vi "数采仪日志报警存储(子VI).vi"   [LabVIEW 2016]
types:
  T1 = cluster{"时间标识":timestamp, "设备":string, "日志信息":string, "流程参数":string}
  T2 = cluster{"时间标识":timestamp, "设备":string, "日志信息":string}
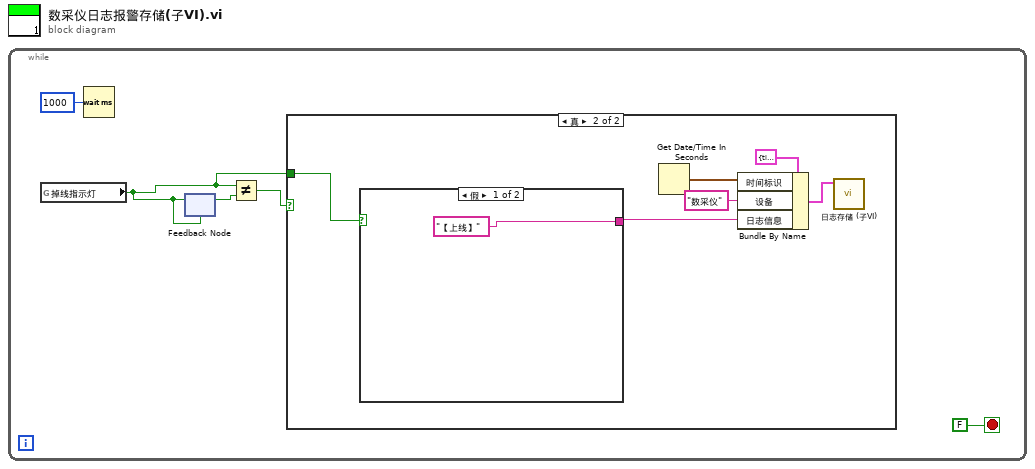
[diagram p0: block diagram]
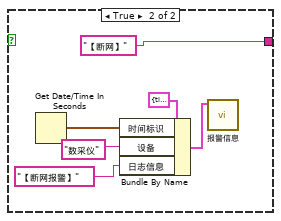
[diagram p3: hidden frame]
diagram:
  n1 = while {
    stop <- FALSE stop-if-true
    n2 = global read "全局 数据发送重叠.vi" "掉线指示灯"() -> (w1:bool)
    n3 = Wait (ms)(milliseconds to wait=u32 1000 ("等待时间（毫秒）")) -> ()  [unwired: 1 out]
    n4 = feedback-in #1(w1) -> ()
    n5 = feedback #1(w1) -> (w3:bool)
    n6 = Not Equal?(x=w1, y=w3) -> (x != y?=w2:bool)
    n7 = case shown="真" w2 {
      tunnel: w1 -> [_ w6]
      frame False {
      }
      frame True {
        n8 = case shown="假" w6 {
          tunnel: ["【上线】" ("设备") "【断网】" ("设备")] -> w7
          frame False {
          }
          frame True {
            n9 = Get Date/Time In Seconds() -> (seconds since 1Jan1904=w15:timestamp)
            n10 = Bundle By Name(cluster=T2 {"时间标识"=timestamp(0 s since 1904-01-01), "设备"="", "日志信息"=""} ("data in"), "时间标识"=w15, "设备"="数采仪", "日志信息"="【断网报警】" ("设备")) -> (w16:T2)
            n11 = call "报警信息.vi"("data in"=w16) -> ()  [unwired: 10 in, 1 out]
          }
        }
        n12 = Get Date/Time In Seconds() -> (seconds since 1Jan1904=w9:timestamp)
        n13 = Bundle By Name(cluster=T1 {"时间标识"=timestamp(0 s since 1904-01-01), "设备"="", "日志信息"="", "流程参数"=""} ("data in"), "时间标识"=w9, "设备"="数采仪", "日志信息"=w7) -> (w10:T1)
        n14 = call "日志存储 (子VI).vi"("data in"=w10) -> ()  [unwired: 11 in]
      }
    }
  }
